vi "DP-Config.vi"(0 "StimGen":T1, 1 "DP Freqs":T3, 5 "DataAcq":T2, 11 "error in (no error)":errorcluster) -> (6 "AO Channels":i32[](array[numeric]), 15 "error out":errorcluster)   [LabVIEW 2020]
uses:
  Typedefs/DP-Freqs.ctl
  Typedefs/DP-DataAcq.ctl
  Typedefs/DP-StimGen.ctl
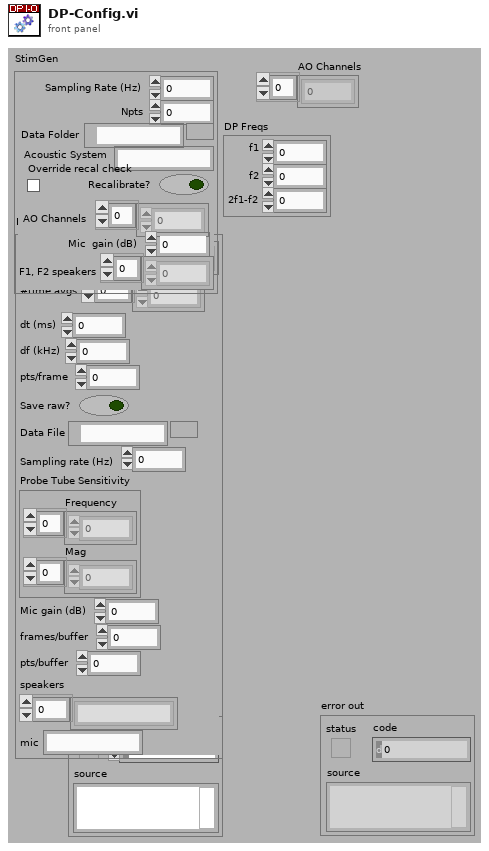
[diagram p1: front panel]
types:
  T1 = typedef "DP-StimGen.ctl" = cluster{"Sampling Rate (Hz)":dbl, "Npts":i32, "Data Folder":path, "Acoustic System":string, "Recalibrate?":bool, "AO Channels":i32[], "Mic  gain (dB)":dbl, "F1, F2 speakers":i32[], "Override recal check":bool}
  T2 = typedef "DP-DataAcq.ctl" = cluster{"#spectra avgs":i32[], "#time avgs":i32[], "dt (ms)":dbl, "df (kHz)":dbl, "pts/frame":i32, "Save raw?":bool, "Data File":path, "Sampling rate (Hz)":dbl, "Probe Tube Sensitivity":cluster{"Frequency":dbl[], "Mag":dbl[]}, "Mic gain (dB)":dbl, "frames/buffer":i32, "pts/buffer":i32, "speakers":string[], "mic":string}
  T3 = typedef "DP-Freqs.ctl" = cluster{"f1":dbl, "f2":dbl, "2f1-f2":dbl}
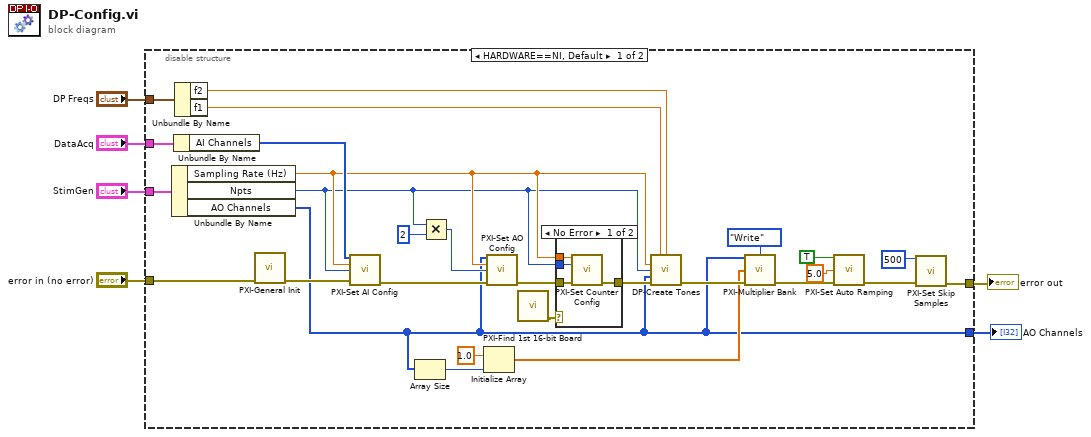
[diagram p0: block diagram]
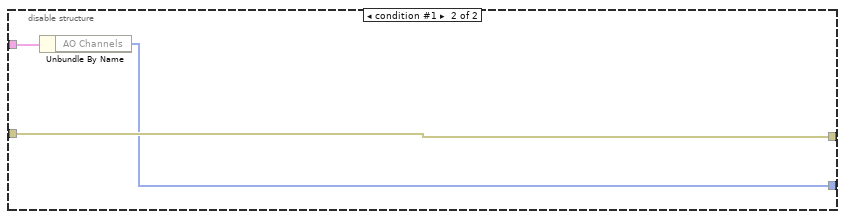
[diagram p3: hidden frame]
diagram:
  n1 = disable-structure shown="HARDWARE==NI, Default" {
    disable-tunnel: "error in (no error)" -> [w33 w42]
    disable-tunnel: "StimGen" -> [w22 w41]
    disable-tunnel: "DataAcq" -> [w21 _]
    disable-tunnel: "DP Freqs" -> [w19 _]
    disable-tunnel: [w12 w42] -> w2
    disable-tunnel: [w8 w40] -> w1
    frame condition #0 (active) {
      n2 = Unbundle By Name(w22) -> ("Sampling Rate (Hz)"=w10:dbl, "Npts"=w9:i32, "AO Channels"=w8:i32[])
      n3 = Unbundle By Name(w21) -> ("AI Channels"=w20:u16[])
      n4 = Unbundle By Name(w19) -> ("f2"=w17:dbl, "f1"=w18:dbl)
      n5 = call "PXI-General Init.vi"("error in (no error)"=w33) -> ("error out"=w31:errorcluster)  [unwired: 10 in]
      n6 = call "PXI-Set AI Config.vi"("AI Channels"=w20, "Sampling Rate (Hz)"=w10, "Buffer Size"=w9, "error in (no error)"=w31) -> ("error out"=w30:errorcluster)  [unwired: 11 in]
      n7 = Array Size(array=w8) -> (size(s)=w26:i32)
      n8 = Multiply(x=w9, y=2) -> (x*y=w29:i32)
      n9 = Initialize Array(1.0 ("element"), w26) -> (w24:dbl[])
      n10 = call "PXI-Set AO Config.vi"("AO Channels"=w8, "Sampling Rate (Hz)"=w10, "Buffer Size"=w29, "error in (no error)"=w30) -> ("error out"=w11:errorcluster)  [unwired: 11 in]
      n11 = call "PXI-Find 1st 16-bit Board.vi"() -> ("error out"=w7:errorcluster)  [unwired: 9 in, 2 out]
      n12 = case shown="No Error" w7 {
        tunnel: [w38 w39] -> w34
        tunnel: w11 -> [w37 w39]
        tunnel: w10 -> [w36 _]
        tunnel: w9 -> [w35 _]
        frame No Error {
          n13 = call "PXI-Set Counter Config.vi"("AI Sampling Rate (Hz)"=w36, "Num AI Pts"=w35, "error in (no error)"=w37) -> ("error out"=w38:errorcluster)  [unwired: 12 in]
        }
        frame Error {
        }
      }
      n14 = call "DP-Create Tones.vi"("f1"=w18, "f2"=w17, "Sampling rate (Hz)"=w10, "Npts"=w9, "AO channels"=w8, "error in (no error)"=w34) -> ("error out"=w28:errorcluster)  [unwired: 8 in, 1 out]
      n15 = call "PXI-Multiplier Bank.vi"("AO Channels"=w8, "Action"=enum16{"Init", "Write", "Read"}."Write", "Multipliers"=w24, "error in (no error)"=w28) -> ("error out"=w27:errorcluster)  [unwired: 9 in, 2 out]
      n16 = call "PXI-Set Auto Ramping.vi"("Auto ramp?"=TRUE ("Ramp up?"), "Ramp duration (ms)"=5.0, "error in (no error)"=w27) -> ("error out"=w14:errorcluster)  [unwired: 12 in]
      n17 = call "PXI-Set Skip Samples.vi"("Number of samples to skip (-1)"=500 ("Skip Samples"), "error in (no error)"=w14) -> ("error out"=w12:errorcluster)  [unwired: 13 in]
    }
    frame condition #1 {
      n18 = Unbundle By Name(w41) -> ("AO Channels"=w40:i32[])
    }
  }
  "error out" <- w2
  "AO Channels" <- w1
